vi "Generate Address.vi"(8 "error in (no error)":errorcluster, 11 "7-Bit in":refnum<class "7-Bit.lvclass">) -> (0 "error out":errorcluster, 3 "7-Bit out":refnum<class "7-Bit.lvclass">)   [LabVIEW 2020, in "7-Bit.lvclass"]
uses:
  7-Bit.lvclass
  C:/Users/kaiser.asan/OneDrive - SolitonTechnologies/LabVIEW/29.SDLC - I2C Driver/I2C Module/I2C Controller Module/Class/Addressing Mode/Parent/Addressing Mode.lvclass
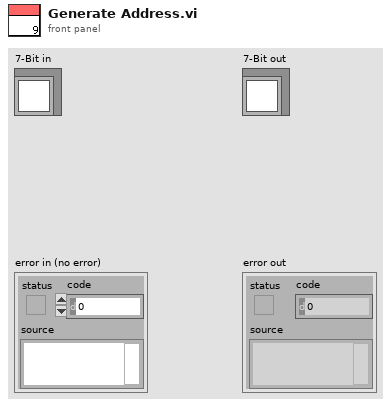
[diagram p1: front panel]
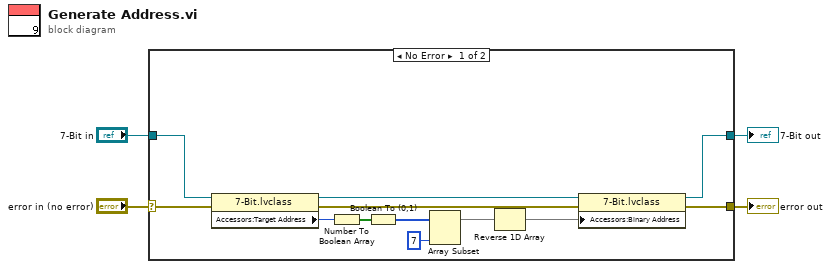
[diagram p0: block diagram]
diagram:
  n1 = case shown="No Error" "error in (no error)" {
    selector: "error in (no error)" -> [w16 w18]
    tunnel: [w11 w18] -> w4
    tunnel: [w8 w17] -> w3
    tunnel: "7-Bit in" -> [w14 w17]
    frame No Error {
      n2 = property class="7-Bit.lvclass"(reference=w14, error in=w16) -> (reference out=w10:refnum<class "7-Bit.lvclass">, error out=w15:errorcluster, "Accessors:Target Address"=w13:u16)
      n3 = Number To Boolean Array(number=w13) -> (Boolean array=w12:bool[])
      n4 = Boolean To (0,1)(Boolean=w12) -> (0, 1=w9:i16[])
      n5 = Array Subset(array=w9, length=7) -> (w6:i16[])  [unwired: 1 in]
      n6 = Reverse 1D Array(array=w6) -> (reversed array=w7:i16[])
      n7 = property class="7-Bit.lvclass"(reference=w10, error in=w15, "Accessors:Binary Address"=w7) -> (reference out=w8:refnum<class "7-Bit.lvclass">, error out=w11:errorcluster)
    }
    frame Error {
    }
  }
  "error out" <- w4
  "7-Bit out" <- w3
